vi "Test Submit.vi"(0 "Export in":refnum<class "Export.lvclass">) -> (4 "Export out":refnum<class "Export.lvclass">, 6 "Read for Submit":bool)   [LabVIEW 2017, in "CL_G3_VIComponentBuilder.lvlib" / "Export.lvclass"]
doc: "Calls the comitt behavior's test to see if this export is ready for submission."
uses:
  Export.lvclass
  Export.lvclass/Export.ctl
  Commit Behavior/Commit/Commit.lvclass/Commit.ctl
  Accessors/Read Commit behavior.vi
  Commit Behavior/Commit/Accessors/Read Commit Operation Errors.vi
  Accessors/Write Commit behavior.vi
  Accessors/Write Export Operation Errors.vi
  Commit Behavior/Commit/Commit.lvclass
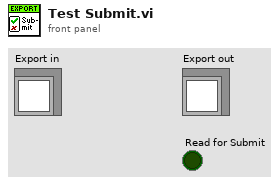
[diagram p1: front panel]
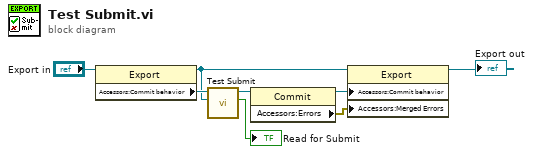
[diagram p0: block diagram]
diagram:
  n1 = property class="Export"(reference="Export in") -> (reference out=w1:refnum<class "Export.lvclass">, "Accessors:Commit behavior"=w4:refnum<class "Commit.lvclass">)  [unwired: 1 in, 1 out]
  n2 = call-dynamic "Test Submit.vi"("Export in"=w1, "Commit in"=w4) -> ("Ready for Submit"=→"Read for Submit":bool, "Commit out"=w3:refnum<class "Commit.lvclass">)  [unwired: 8 in]
  n3 = property class="Commit"(reference=w3) -> (reference out=w6:refnum<class "Commit.lvclass">, "Accessors:Errors"=w2:errorcluster)  [unwired: 1 in, 1 out]
  n4 = property class="Export"(reference=w1, "Accessors:Commit behavior"=w6, "Accessors:Merged Errors"=w2) -> (reference out=→"Export out":refnum<class "Export.lvclass">)  [unwired: 1 in, 1 out]
